vi "CANTEST.vi"(6 "Data Input(Hex)":string="000007d100000000", 8 "错误输入":errorcluster caption="错误输入（无错误）", 9 "ID(Hex 高位有效)":string="00000182", 10 "CANChannel":u32) -> (0 "错误输出":errorcluster, 1 "ErrorSource":string, 3 "帧数据":string)   [LabVIEW 2013]
uses:
  InitConfig.ctl
  DevType.ctl
panel:
  out "Result":bool
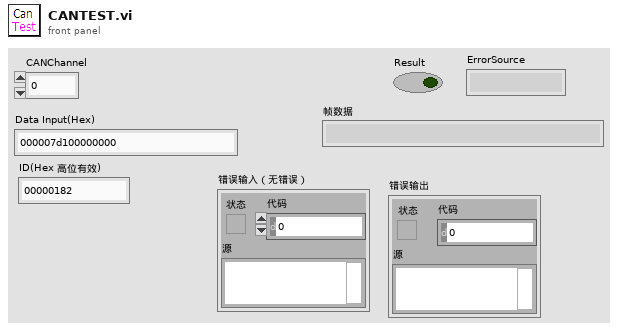
[diagram p1: front panel]
types:
  T1 = typedef "DevType.ctl" = u16
  T2 = typedef "InitConfig.ctl" = cluster{"AccCode":u32, "AccMask":u32, "Reserved":u32, "Filter":u8, "kCanBaud":u8, "Timing0":u8, "Timing1":u8, "Mode":u8, "CanRx_IER":u8}
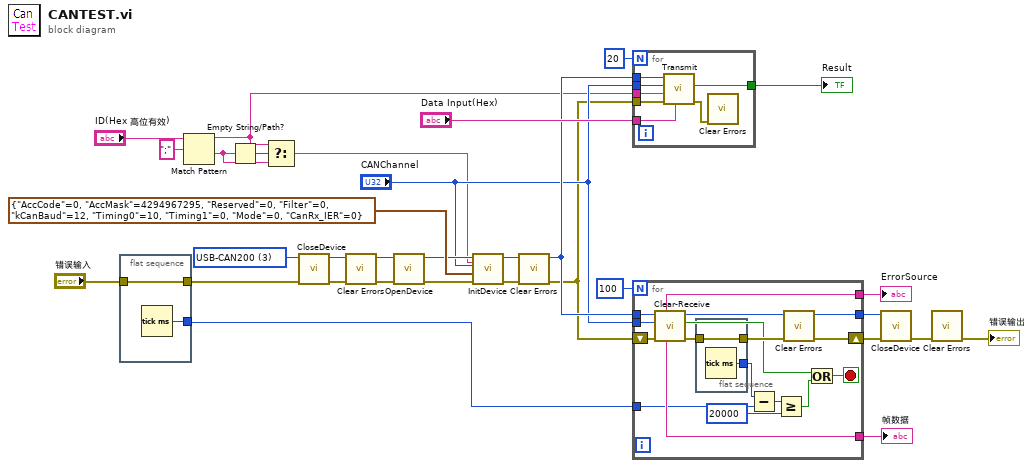
[diagram p0: block diagram]
diagram:
  w29 = T1 3 items=["PCI-CAN200"=7, "USB-CAN"=2, "USB-CAN200"=3] ("DeviceType")
  n1 = flat-sequence {
    tunnel: [w32] -> w7
    tunnel: "错误输入" -> [w32]
    tunnel: [w31] -> w4
    frame #0 {
      n2 = Tick Count (ms)() -> (millisecond timer value=w31:u32)
    }
  }
  n3 = Match Pattern(string="ID(Hex 高位有效)", regular expression=";" ("正则表达式")) -> (before substring=w10:string, after substring=w9:string)  [unwired: 1 in, 2 out]
  n4 = Empty String/Path?(string/path=w9) -> (empty?=w11:bool)
  n5 = Select(t=w10, s=w11, f=w9) -> (s? t:f=w8:string)
  n6 = call "CloseDevice.vi"("错误输入（无错误）"=w7, "DeviceType"=w29) -> ("错误输出"=w23:errorcluster, "DeviceTypeOut"=w28:u16)  [unwired: 7 in, 1 out]
  n7 = call <vilib>:"Clear Errors.vi"("error in (no error)"=w23) -> ("error out"=w5:errorcluster)  [unwired: 6 in]
  n8 = call "OpenDevice.vi"("错误输入（无错误）"=w5, "DeviceType"=w28) -> ("错误输出"=w24:errorcluster, "DeviceTypeOut"=w27:u16)  [unwired: 7 in, 1 out]
  n9 = call "InitDevice.vi"("ID(Hex 高位有效)"=w8, "错误输入（无错误）"=w24, "InitConfig"=T2 {"AccCode"=0, "AccMask"=4294967295, "Reserved"=0, "Filter"=0, "kCanBaud"=12, "Timing0"=10, "Timing1"=0, "Mode"=0, "CanRx_IER"=0}, "CanChannel"="CANChannel", "DeviceType"=w27) -> ("错误输出"=w19:errorcluster, "DeviceTypeOut"=w16:u16)  [unwired: 4 in, 1 out]
  n10 = call <vilib>:"Clear Errors.vi"("error in (no error)"=w19) -> ("error out"=w2:errorcluster)  [unwired: 6 in]
  n11 = for {
    N: 20 -> [_]
    tunnel: [w39] -> w26
    tunnel: w10 -> [w38]
    tunnel: "Data Input(Hex)" -> [w37]
    tunnel: "CANChannel" -> [w36]
    tunnel: w2 -> [w35]
    tunnel: w16 -> [w34]
    n12 = call "Transmit.vi"("Data Input(Hex)"=w37, "错误输入（无错误）"=w35, "ID(Hex 高位有效)"=w38, "CANChannel"=w36, "DeviceType"=w34) -> ("错误输出"=w33:errorcluster, "Result"=w39:bool)  [unwired: 4 in, 1 out]
    n13 = call <vilib>:"Clear Errors.vi"("error in (no error)"=w33) -> ()  [unwired: 6 in, 1 out]
  }
  "Result" <- w26
  n14 = for {
    N: 100 -> [_]
    tunnel: "CANChannel" -> [w55]
    tunnel: [w53] -> w18
    tunnel: w16 -> [w52]
    tunnel: [w51] -> w17
    shift-right: [w46] -> w20
    shift-left: w2 -> [w54]
    tunnel: w4 -> [w47]
    tunnel: [w40] -> w1
    stop <- w41 stop-if-true
    n15 = call "Clear-Receive.vi"("错误输入"=w54, "CANChannel"=w55, "DeviceType"=w52) -> ("错误输出"=w50:errorcluster, "Result"=w43:bool, "DeviceTypeOut"=w51:u16, "data"=w53:string, "ErrorSource"=w40:string)  [unwired: 1 in, 3 out]
    n16 = flat-sequence {
      tunnel: w50 -> [w57]
      tunnel: [w57] -> w49
      tunnel: [w56] -> w48
      frame #0 {
        n17 = Tick Count (ms)() -> (millisecond timer value=w56:u32)
      }
    }
    n18 = Subtract(x=w48, y=w47) -> (x-y=w45:u32)
    n19 = Greater Or Equal?(x=w45, y=20000) -> (x >= y?=w42:bool)
    n20 = call <vilib>:"Clear Errors.vi"("error in (no error)"=w49) -> ("error out"=w46:errorcluster)  [unwired: 6 in]
    n21 = Or(x=w43, y=w42) -> (x .or. y?=w41:bool)
  }
  "帧数据" <- w18
  "ErrorSource" <- w1
  n22 = call "CloseDevice.vi"("错误输入（无错误）"=w20, "DeviceType"=w17) -> ("错误输出"=w22:errorcluster)  [unwired: 7 in, 2 out]
  n23 = call <vilib>:"Clear Errors.vi"("error in (no error)"=w22) -> ("error out"=→"错误输出":errorcluster)  [unwired: 6 in]
